vi "Globals.vi"() -> ()   [LabVIEW 2020, in "2021_12.lvclass"]
uses:
  2021_12.lvclass
  12_Cave_class/12_Cave.lvclass
panel:
  in  "Paths":T1(array[cluster])
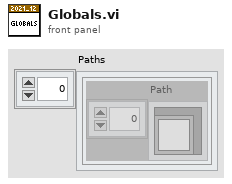
[diagram p1: front panel]
types:
  T1 = cluster{"Path":refnum<class "12_Cave.lvclass">[]}[]
diagram:
